vi "Using Temperature.vi"() -> ()   [LabVIEW 2012]
panel:
  in  "停止按钮":bool
  out "图表":dbl(graph)
  in  "延迟乘数":dbl(knob) min=0.0 max=2.0 step=0.1 scale=0.0..2.0
  in  "数值":i32
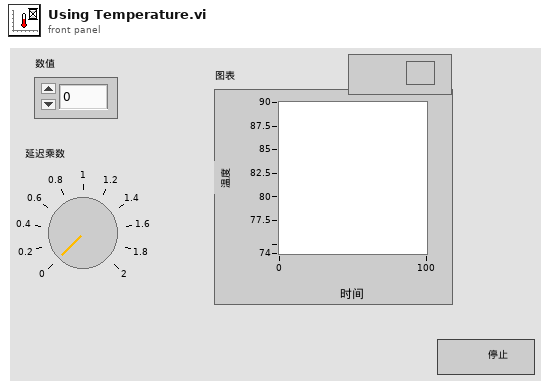
[diagram p1: front panel]
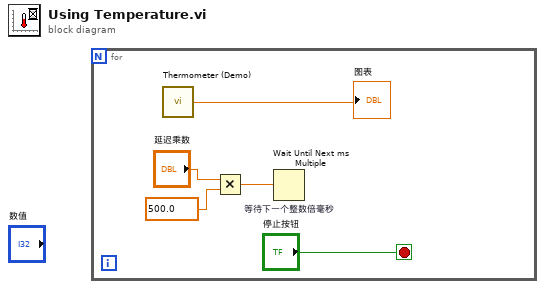
[diagram p0: block diagram]
diagram:
  n1 = for {
    stop <- "停止按钮" stop-if-true
    n2 = call "Thermometer (Demo).vi"() -> ("温度值"=→"图表":dbl)  [unwired: 1 in]
    n3 = Multiply ("乘")(x="延迟乘数", y=500.0) -> (x*y=w3:dbl)
    n4 = Wait Until Next ms Multiple "等待下一个整数倍毫秒"(millisecond multiple=w3) -> ()  [unwired: 1 out]
  }
